vi "PathPlanner_Trajectory_GenerateStates_Pass2.vi"(11 "in PathPlannerStates":T1[](array[typedef]) {"TargetHolonomicRotation"."SIN" format="%13.4f"; "TargetHolonomicRotation"."COS" format="%13.4f"; "TargetHolonomicRotation"."VALUE" format="%13.4f"; "Heading"."SIN" format="%13.4f"; "Heading"."COS" format="%13.4f"; "Heading"."VALUE" format="%13.4f"; "PositionMeters"."Y" format="%14.3f"; "PositionMeters"."X" format="%14.3f"}) -> (3 "out PathPlannerStates":T1[](array[typedef]) {"TargetHolonomicRotation"."SIN" format="%13.4f"; "TargetHolonomicRotation"."COS" format="%13.4f"; "TargetHolonomicRotation"."VALUE" format="%13.4f"; "Heading"."SIN" format="%13.4f"; "Heading"."COS" format="%13.4f"; "Heading"."VALUE" format="%13.4f"; "PositionMeters"."Y" format="%14.3f"; "PositionMeters"."X" format="%14.3f"})   [LabVIEW 2019, in "PathPlanner24.lvlib"]
doc: "Internal routine to help create a trajectory from a path."
uses:
  PathPlanner24.lvlib
  TypeDef/PathPlannerTrajectoryState.ctl
  <vilib>/Rock Robotics/WPI/ThirdParty/JAS_Junk/TrajLib/TypeDef/TRANSLATION2D.ctl
  <vilib>/Rock Robotics/WPI/ThirdParty/JAS_Junk/TrajLib/TypeDef/ROTATION2D.ctl
  TypeDef/PathPlannerPathConstraints.ctl
  <vilib>/Rock Robotics/WPI/ThirdParty/JAS_Junk/TrajLib/Trajectory_Library.lvlib
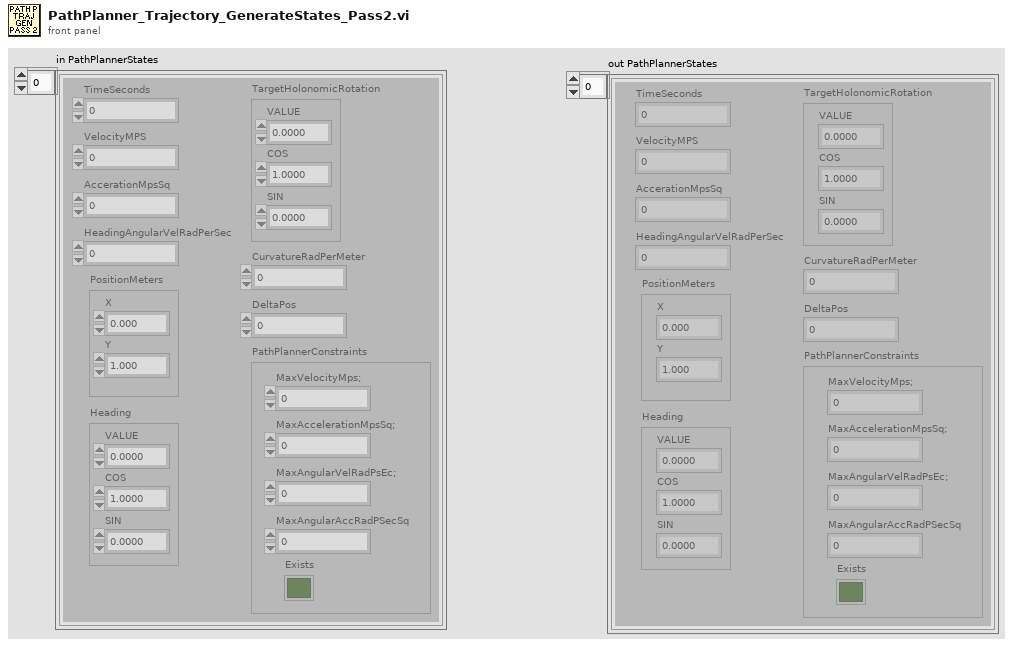
[diagram p1: front panel]
types:
  T1 = typedef "PathPlanner24.lvlib/PathPlannerTrajectoryState.ctl" = cluster{"TimeSeconds":dbl, "VelocityMPS":dbl, "AccerationMpsSq":dbl, "HeadingAngularVelRadPerSec":dbl, "PositionMeters":T2, "Heading":T3, "TargetHolonomicRotation":T3, "CurvatureRadPerMeter":dbl, "PathPlannerConstraints":T4, "DeltaPos":dbl}
  T2 = typedef "Trajectory_Library.lvlib/TRANSLATION2D.ctl" = cluster{"X":dbl, "Y":dbl}
  T3 = typedef "Trajectory_Library.lvlib/ROTATION2D.ctl" = cluster{"VALUE":dbl, "COS":dbl, "SIN":dbl}
  T4 = typedef "PathPlanner24.lvlib/PathPlannerPathConstraints.ctl" = cluster{"MaxVelocityMps;":dbl, "MaxAccelerationMpsSq;":dbl, "MaxAngularVelRadPsEc;":dbl, "MaxAngularAccRadPSecSq":dbl, "Exists":bool}
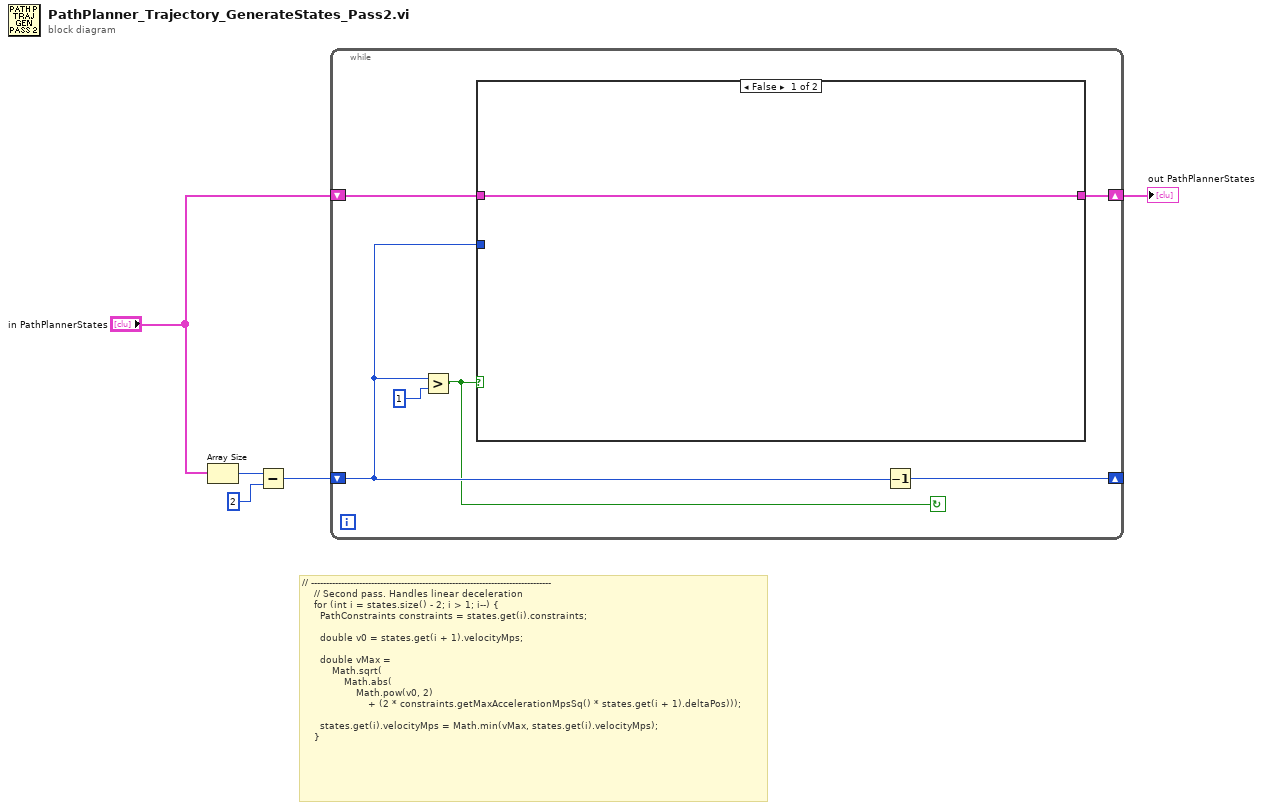
[diagram p0: block diagram]
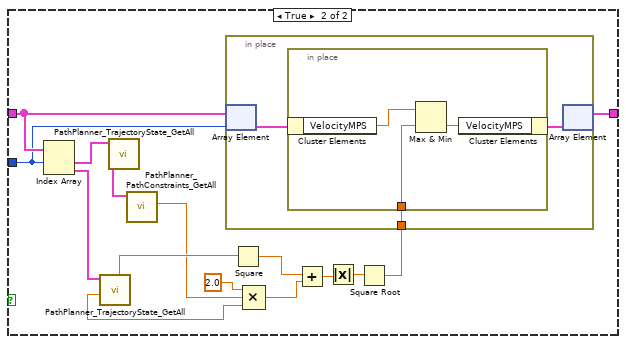
[diagram p2: hidden frame]
diagram:
  # "// --------------------------------------------------------------------------------\n    // Second pass. Handles linear deceleration\n    for (int i = states.size() - 2; i > 1; i--) {\n      PathConstraints constraints = states.get(i).constraints;\n\n      double v0 = states.get(i + 1).velocityMps;\n\n      double vMax =\n          Math.sqrt(\n              Math.abs(\n                  Math.pow(v0, 2)\n                      + (2 * constraints.getMaxAccelerationMpsSq() * states.get(i + 1).deltaPos)));\n\n      states.get(i).velocityMps = Math.min(vMax, states.get(i).velocityMps);\n    }"
  n1 = Array Size(array="in PathPlannerStates") -> (size(s)=w5:i32)
  n2 = Subtract(x=w5, y=2) -> (x-y=w3:i32)
  n3 = while {
    shift-right: [w11] -> _
    shift-left: w3 -> [w8]
    shift-right: [w9] -> w1
    shift-left: "in PathPlannerStates" -> [w10]
    stop <- w6 continue-if-true
    n4 = Greater?(x=w8, y=1) -> (0:w6:bool)
    n5 = case shown="False" w6 {
      tunnel: w10 -> [w12 w25]
      tunnel: w8 -> [_ w24]
      tunnel: [w12 w23] -> w9
      frame False {
      }
      frame True {
        n6 = Index Array(array=w25, index #1=w24) -> (element #1=w27:T1, element #2=w26:T1)  [unwired: 1 in]
        n7 = call "PathPlanner_TrajectoryState_GetAll.vi"("PathPlannerState"=w26) -> ("VelocityMPS"=w22:dbl, "DeltaPos"=w18:dbl)  [unwired: 1 in, 8 out]
        n8 = call "PathPlanner_TrajectoryState_GetAll.vi"("PathPlannerState"=w27) -> ("PathPlannerConstraints"=w20:T4)  [unwired: 1 in, 9 out]
        n9 = call "PathPlanner_PathConstraints_GetAll.vi"("PathPlannerConstraints"=w20) -> ("MaxAccelerationMpsSq;"=w19:dbl)  [unwired: 6 in, 4 out]
        n10 = Square(x=w22) -> (x^2=w16:dbl)
        n11 = Compound Arithmetic op=MULTIPLY(2.0 ("x"), w19, w18) -> (w17:dbl)
        n12 = Add(x=w16, y=w17) -> (x+y=w15:dbl)
        n13 = Absolute Value(x=w15) -> (abs(x)=w14:dbl)
        n14 = Square Root(x=w14) -> (sqrt(x)=w13:dbl)
        n15 = in-place {
          in-place-border: w13 -> [w28]
          n16 = in-place-array #1(w25, w24) -> (w30:T1)
          n17 = in-place {
            in-place-border: w28 -> [w31]
            n18 = in-place-cluster #2(w30) -> ("VelocityMPS"=w32:dbl)
            n19 = Max & Min(x=w32, y=w31) -> (min(x,y)=w33:dbl)  [unwired: 1 out]
            n20 = in-place-cluster #2("VelocityMPS"=w33) -> (w29:T1)
          }
          n21 = in-place-array #1(w29) -> (w23:T1[])  [unwired: 1 out]
        }
      }
    }
    n22 = Decrement(x=w8) -> (x-1=w11:i32)
  }
  "out PathPlannerStates" <- w1
